vi "Helper SubVI - Configure Bispectrum Indicator.vi"(7 "display all? (T)":bool=TRUE, 8 "error in (no error)":errorcluster, 10 "frequency bins":dbl[](array[numeric]), 11 "S(f,f)":dbl[][](array[numeric])) -> (0 "error out":errorcluster, 3 "bispectrum  indicator":refnum<class "Base Datatype.lvclass">[](xcontrol))   [LabVIEW 2023]
doc: "Configures and displays the bispectrum of a univariate time series."
uses:
  <vilib>/Native 3D Graph/xcontrol/3DPC_SurfacePlot.xctl
  <vilib>/Native 3D Graph/classes/Base Datatype.lvclass
  <vilib>/addons/_Advanced Signal Processing/NI_AdvSigProcTSA.lvlib
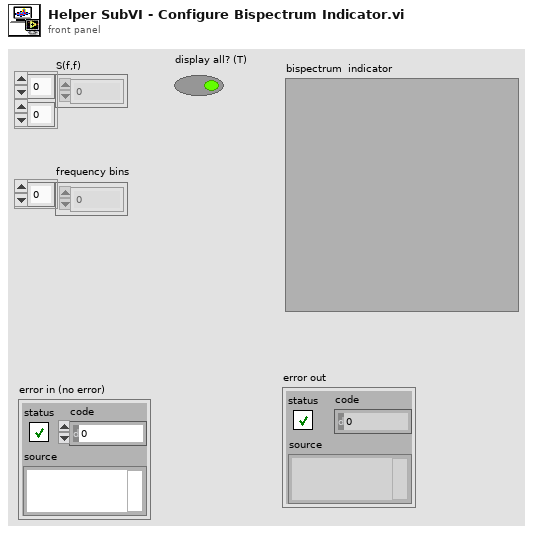
[diagram p1: front panel]
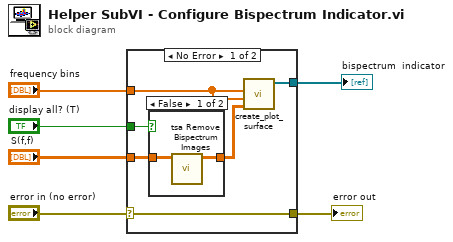
[diagram p0: block diagram]
diagram:
  n1 = case shown="No Error" "error in (no error)" {
    selector: "error in (no error)" -> [w10 w16]
    tunnel: "S(f,f)" -> [w11 _]
    tunnel: "frequency bins" -> [w8 _]
    tunnel: [w10 w16] -> w4
    tunnel: "display all? (T)" -> [w12 _]
    tunnel: [w7 _] -> w1
    frame No Error {
      n2 = case shown="False" w12 {
        tunnel: w11 -> [w14 w15]
        tunnel: [w13 w15] -> w9
        frame False {
          n3 = call <vilib>:"tsa Remove Bispectrum Images.vi"("bispectrum in"=w14) -> ("bispectrum out"=w13:dbl[][])  [unwired: 10 in]
        }
        frame True {
        }
      }
      n4 = call <vilib>:"create_plot_surface.vi"("z matrix"=w9, "y vector"=w8, "x vector"=w8) -> ("plots out"=w7:refnum<class "Base Datatype.lvclass">[])  [unwired: 2 in, 6 out]
    }
    frame Error {
    }
  }
  "error out" <- w4
  "bispectrum  indicator" <- w1
